vi "makepath.vi"(8 "end":dbl[](array[numeric]), 11 "start":dbl[](array[numeric])) -> (3 "out":dbl[](array[numeric]))   [LabVIEW 2015]
panel:
  out "b":dbl
  out "a":dbl
  out "y'":dbl
  out "y":dbl
  out "x":dbl
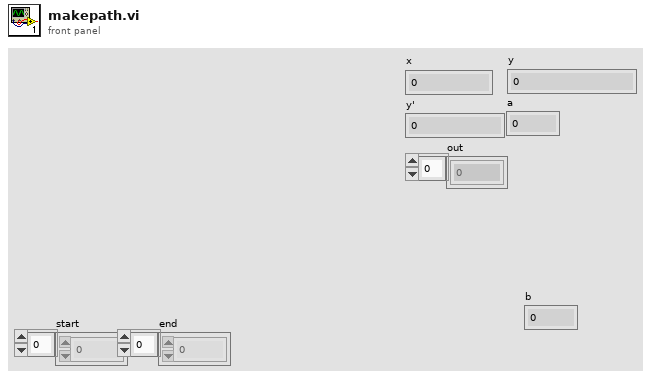
[diagram p1: front panel]
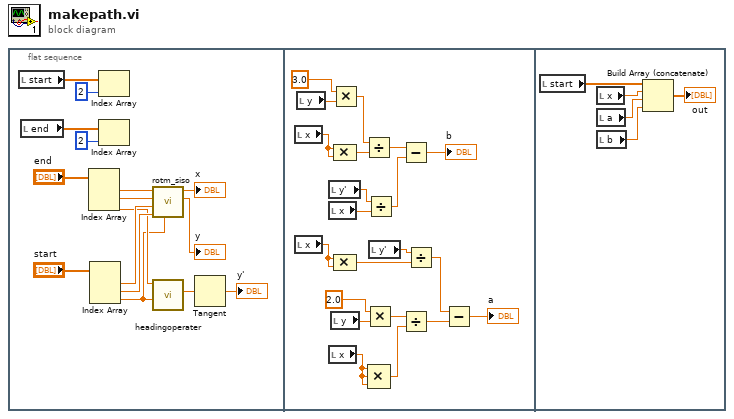
[diagram p0: block diagram]
diagram:
  n1 = flat-sequence {
    frame #0 {
      n2 = local read "start"() -> (w5:dbl[])
      n3 = local read "end"() -> (w8:dbl[])
      n4 = Index Array(array="end") -> (element #1=w12:dbl, element #2=w11:dbl, element #3=w4:dbl)  [unwired: 3 in]
      n5 = Index Array(array="start") -> (element #1=w15:dbl, element #2=w14:dbl, element #3=w3:dbl)  [unwired: 3 in]
      n6 = Index Array(array=w5, index=2) -> ()  [unwired: 1 out]
      n7 = Index Array(array=w8, index=2) -> ()  [unwired: 1 out]
      n8 = call "rotm_siso.vi"("angle[rad]"=w3, "y0"=w14, "x0"=w15, "y"=w11, "x"=w12) -> ("y'"=→"y":dbl, "x'"=→"x":dbl)  [unwired: 5 in]
      n9 = call "headingoperater.vi"("h1"=w3, "h2"=w4) -> ("h2-h1"=w2:dbl)  [unwired: 8 in, 1 out]
      n10 = Tangent(1:w2) -> (0:→"y'":dbl)
    }
    frame #1 {
      n11 = local read "x"() -> (w20:dbl)
      n12 = local read "x"() -> (w30:dbl)
      n13 = local read "y"() -> (w22:dbl)
      n14 = local read "y'"() -> (w25:dbl)
      n15 = local read "x"() -> (w18:dbl)
      n16 = local read "x"() -> (w37:dbl)
      n17 = Multiply(x=3.0 ("value"), y=w22) -> (x*y=w23:dbl)
      n18 = local read "y"() -> (w35:dbl)
      n19 = Compound Arithmetic op=MULTIPLY(w20, w20) -> (w24:dbl)
      n20 = Compound Arithmetic op=MULTIPLY(w30, w30) -> (w32:dbl)
      n21 = Divide(x=w23, y=w24) -> (x/y=w19:dbl)
      n22 = Multiply(x=2.0 ("value"), y=w35) -> (x*y=w34:dbl)
      n23 = Divide(x=w25, y=w18) -> (x/y=w17:dbl)
      n24 = Compound Arithmetic op=MULTIPLY(w37, w37, w37) -> (w33:dbl)
      n25 = local read "y'"() -> (w31:dbl)
      n26 = Subtract(x=w19, y=w17) -> (x-y=→"b":dbl)
      n27 = Divide(x=w34, y=w33) -> (x/y=w28:dbl)
      n28 = Divide(x=w31, y=w32) -> (x/y=w29:dbl)
      n29 = Subtract(x=w29, y=w28) -> (x-y=→"a":dbl)
    }
    frame #2 {
      n30 = local read "start"() -> (w42:dbl[])
      n31 = local read "x"() -> (w41:dbl)
      n32 = local read "a"() -> (w40:dbl)
      n33 = local read "b"() -> (w39:dbl)
      n34 = Build Array (concatenate)(w42, w41, w40, w39) -> (→"out":dbl[])
    }
  }
